vi "Configure Parallel.vi"(0 "VISA resource name":refnum<visa-resource-name>, 5 "Auxiliaries IP LSBs":u16[](array[numeric]), 11 "error in (no error)":errorcluster) -> (4 "VISA resource name out":refnum<visa-resource-name>, 15 "error out":errorcluster)   [LabVIEW 2020, in "NH Research Regenerative Test Series.lvlib"]
doc: "This command sets the parallel configuration. This command is only sent to the module that is to be the master. All modules to be paralleled with the master must be set to static IP and all must be on the same IP subnet as the master. For example, if the master IP is 192.100.27.45, then all auxiliaries must have an IP of 192.100.27.xxx.\n\nThis command uses only the last byte (least significant byte LSB) of the IP address. The auxiliaries full IP is the masters IP subnet plus the auxiliaries IP LSB. If no IPs are set, the Master will dissolve its parallel configuration and will act standalone.\n\nAfter sending this command, Configure Save.vi MUST be sent and ALL modules in the parallel group MUST be power cycled to come up in the parallel mode."
uses:
  NH Research Regenerative Test Series.lvlib
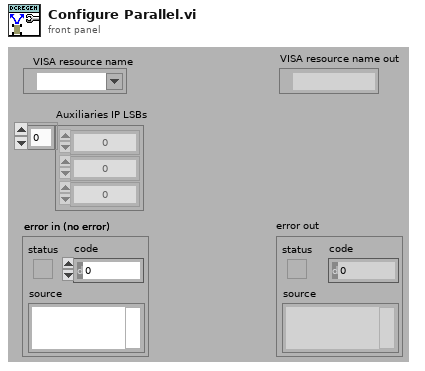
[diagram p1: front panel]
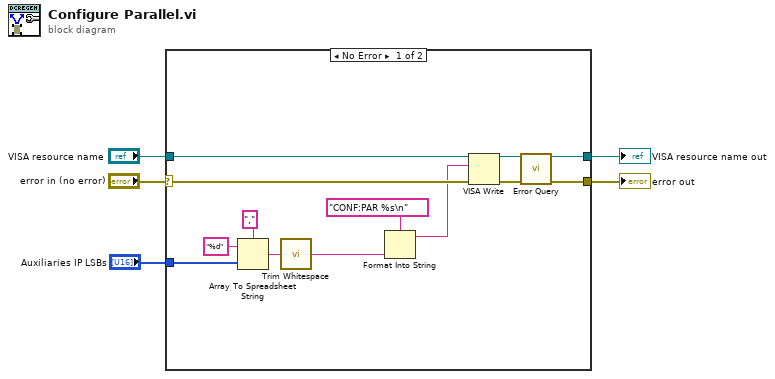
[diagram p0: block diagram]
diagram:
  n1 = case shown="No Error" "error in (no error)" {
    selector: "error in (no error)" -> [w13 w20]
    tunnel: "VISA resource name" -> [w18 w19]
    tunnel: [w17 w19] -> w4
    tunnel: [w16 w20] -> w3
    tunnel: "Auxiliaries IP LSBs" -> [w7 _]
    frame No Error {
      n2 = Array To Spreadsheet String(delimiter (Tab)=",", array=w7, 3:"%d" ("format string")) -> (spreadsheet string=w8:string)
      n3 = call <vilib>:"Trim Whitespace.vi"("string"=w8) -> ("trimmed string"=w6:string)  [unwired: 1 in]
      n4 = Format Into String(format string="CONF:PAR %s\n", w6) -> (resulting string=w11:string)  [unwired: 2 in, 1 out]
      n5 = VISA Write(VISA resource name=w18, write buffer=w11, error in (no error)=w13) -> (VISA resource name out=w15:refnum<visa-resource-name>, error out=w14:errorcluster)  [unwired: 1 out]
      n6 = call "Error Query.vi"("VISA resource name"=w15, "error in (no error)"=w14) -> ("VISA resource name out"=w17:refnum<visa-resource-name>, "error out"=w16:errorcluster)  [unwired: 10 in, 2 out]
    }
    frame Error {
    }
  }
  "error out" <- w3
  "VISA resource name out" <- w4
